vi "CRYCalc Directivity Index.vi"(4 "Weighting curve":string, 6 "Direct_weight":bool caption="Weighting", 7 "Inc(deg.)":i32, 8 "Total Rotation":i32, 9 "Curve Group":string[](array[string]), 10 "Auto Inc":bool caption="Auto Increment", 11 "Curve in":T1={"Name"="", "Curve"=[], "X data"=1, "Y data"=1, "Z data"=1, "X axis"=0, "Y axis"=1, "Z axis"=1, "X unit"="Hz", "Y unit"="", "Z unit"="deg.", "X dB ref"=1.0, "Y dB ref"=1.0, "Z dB ref"=1.0, "single val"=FALSE, "protected"=FALSE, "display X"=TRUE, "display Y"=TRUE, "display Z"=TRUE, "Test Info"="", "Step No."=0, "Plot Settings"={"Color"=0, "Interpolation"=0, "Point Style"=0, "Line Style"=0, "Point Color"=0, "Line Width"=0, "Bar Plot Style"=0, "Fill To"=0}, "AutoProtect"=FALSE} {"Z data" items=["dB", "Lin"]; "X data" items=["dB", "Lin"]; "Y data" items=["dB", "Lin"]; "Z dB ref" format="%.1f"; "Z axis" items=["Log", "Lin"]; "X dB ref" format="%.1f"; "X axis" items=["Log", "Lin"]; "Y axis" items=["Log", "Lin"]; "Y dB ref" format="%.1f"; "Curve"."z" format="%.2f"; "Curve"."y" format="%.2f"; "Curve"."x" format="%.2f"}) -> (3 "Curve out":T1={"Name"="", "Curve"=[], "X data"=1, "Y data"=1, "Z data"=1, "X axis"=0, "Y axis"=1, "Z axis"=1, "X unit"="Hz", "Y unit"="", "Z unit"="deg.", "X dB ref"=1.0, "Y dB ref"=1.0, "Z dB ref"=1.0, "single val"=FALSE, "protected"=FALSE, "display X"=TRUE, "display Y"=TRUE, "display Z"=TRUE, "Test Info"="", "Step No."=0, "Plot Settings"={"Color"=0, "Interpolation"=0, "Point Style"=0, "Line Style"=0, "Point Color"=0, "Line Width"=0, "Bar Plot Style"=0, "Fill To"=0}, "AutoProtect"=FALSE} {"Z data" items=["dB", "Lin"]; "X data" items=["dB", "Lin"]; "Y data" items=["dB", "Lin"]; "Z dB ref" format="%.1f"; "Z axis" items=["Log", "Lin"]; "X dB ref" format="%.1f"; "X axis" items=["Log", "Lin"]; "Y axis" items=["Log", "Lin"]; "Y dB ref" format="%.1f"; "Curve"."z" format="%.2f"; "Curve"."y" format="%.2f"; "Curve"."x" format="%.2f"})   [LabVIEW 2013]
uses:
  Typedef Control/CRYData Cluster.ctl
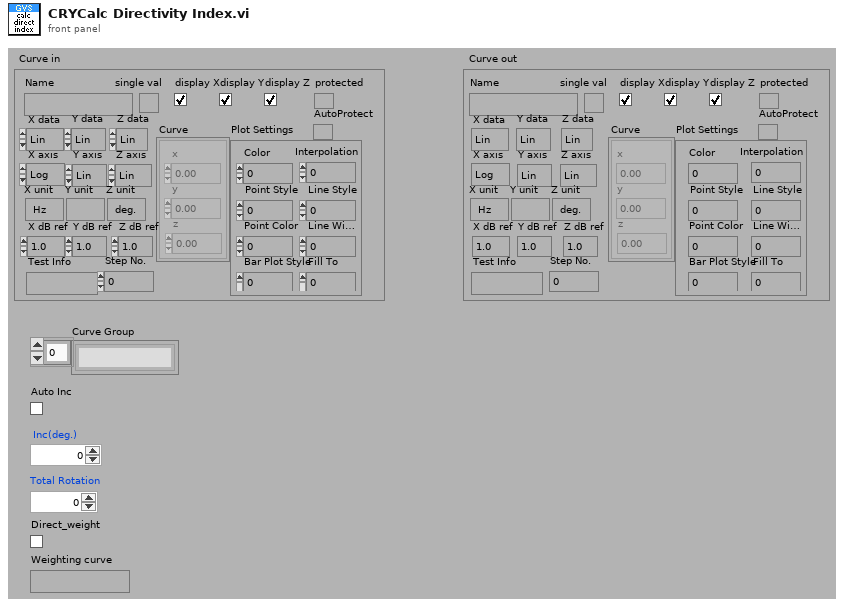
[diagram p1: front panel]
types:
  T1 = typedef "CRYData Cluster.ctl" = cluster{"Name":string, "Curve":cluster{"x":dbl, "y":dbl, "z":dbl}[], "X data":u16, "Y data":u16, "Z data":u16, "X axis":u16, "Y axis":u16, "Z axis":u16, "X unit":string, "Y unit":string, "Z unit":string, "X dB ref":dbl, "Y dB ref":dbl, "Z dB ref":dbl, "single val":bool, "protected":bool, "display X":bool, "display Y":bool, "display Z":bool, "Test Info":string, "Step No.":i32, "Plot Settings":cluster{"Color":u32, "Interpolation":u8, "Point Style":u8, "Line Style":u8, "Point Color":u32, "Line Width":u8, "Bar Plot Style":u8, "Fill To":i16}, "AutoProtect":bool}
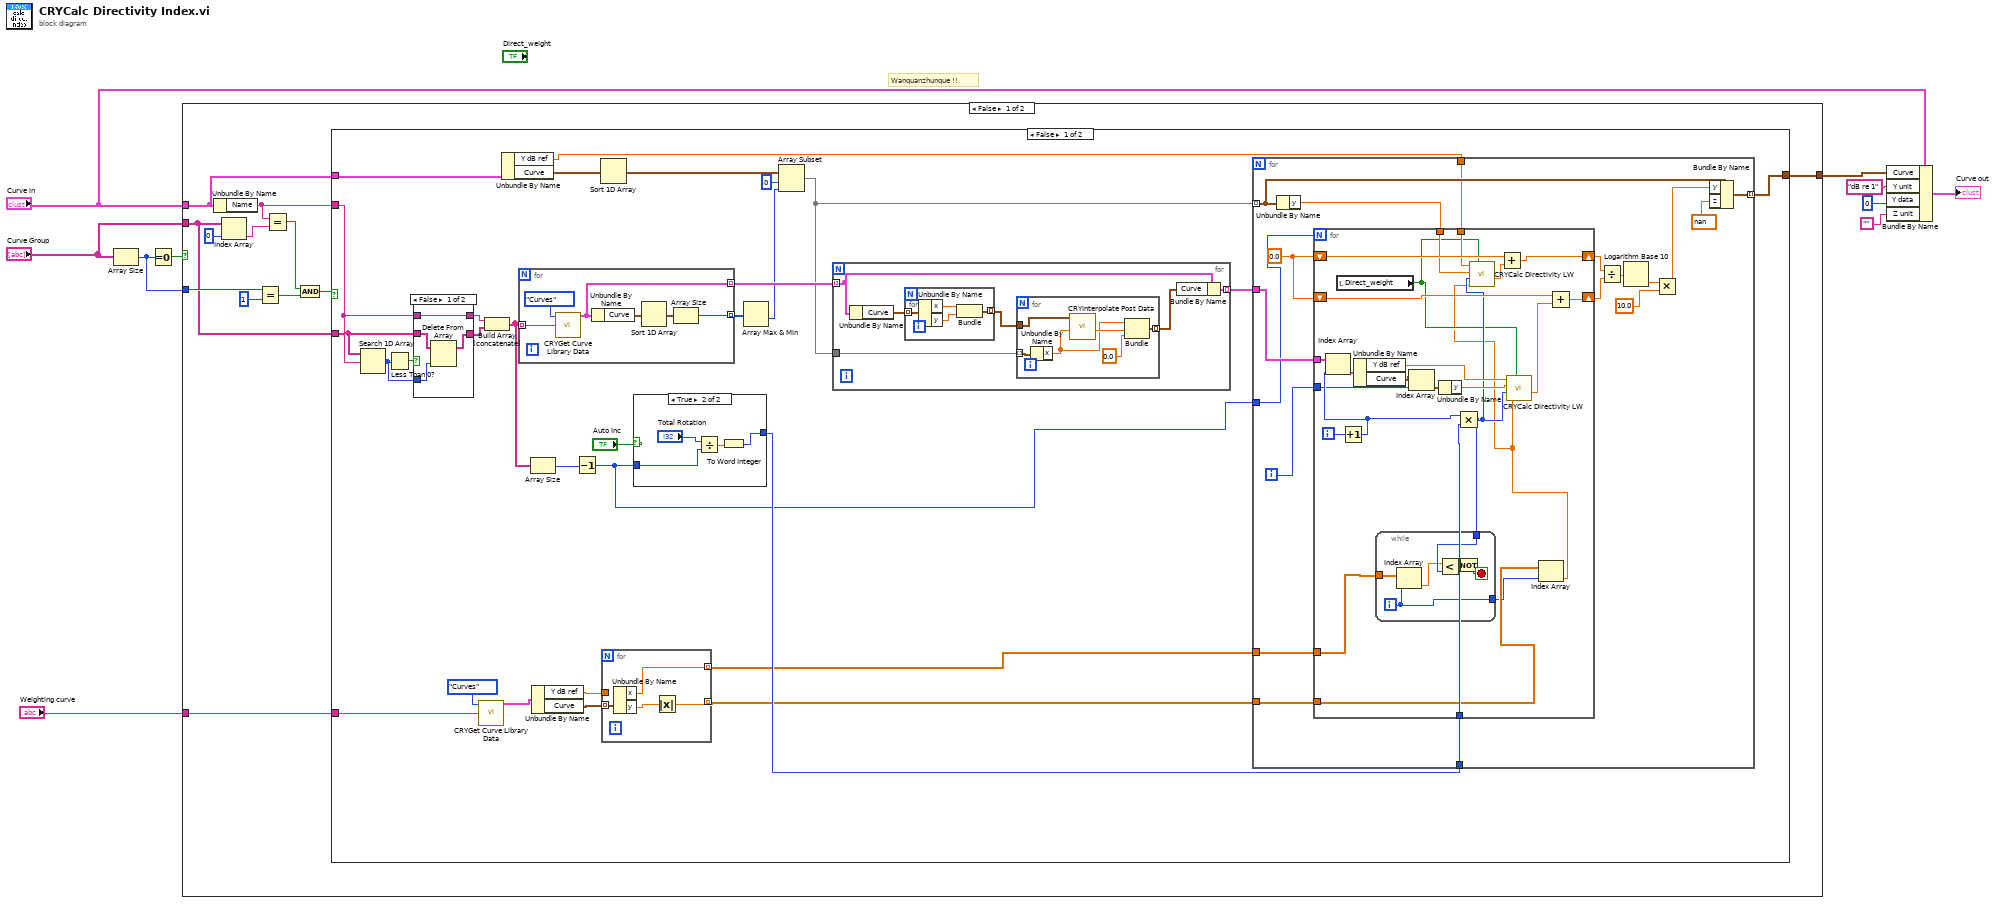
[diagram p0: block diagram]
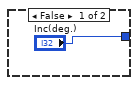
[diagram p2: hidden frame]
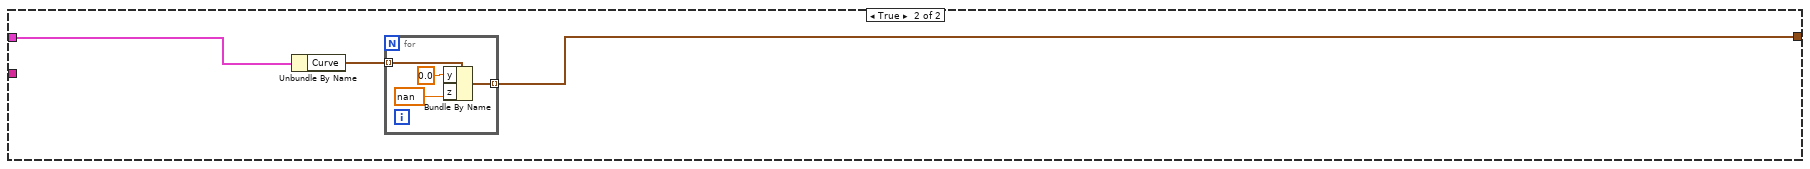
[diagram p4: hidden frame]
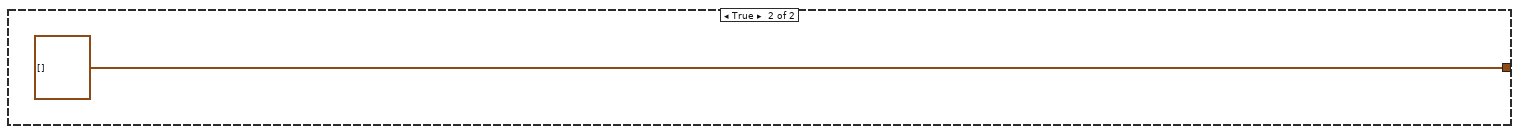
[diagram p5: hidden frame]
diagram:
  # "Wanquanzhunque !!"
  n1 = Array Size(array="Curve Group") -> (size(s)=w5:i32)
  n2 = Equal To 0?(x=w5) -> (x = 0?=w8:bool)
  n3 = case shown="False" w8 {
    tunnel: "Curve in" -> [w17 _]
    tunnel: [w16 cluster{"x":dbl, "y":dbl, "z":dbl}[] [] ("Curve")] -> w6
    tunnel: w5 -> [w22 _]
    tunnel: "Curve Group" -> [w14 _]
    tunnel: "Weighting curve" -> [w11 _]
    frame False {
      n4 = Unbundle By Name(w17) -> ("Name"=w13:string)
      n5 = Index Array(array=w14, index=0) -> (element=w12:string)
      n6 = Equal?(x=w22, y=1) -> (x = y?=w15:bool)
      n7 = Equal?(x=w13, y=w12) -> (x = y?=w19:bool)
      n8 = And(x=w19, y=w15) -> (x .and. y?=w18:bool)
      n9 = case shown="False" w18 {
        tunnel: w17 -> [w51 w139]
        tunnel: [w49 w137] -> w16
        tunnel: w14 -> [w38 _]
        tunnel: w13 -> [w41 _]
        tunnel: w11 -> [w25 _]
        frame False {
          n10 = Search 1D Array(1D array=w38, element=w41) -> (index of element=w37:i32)  [unwired: 1 in]
          n11 = Less Than 0?(x=w37) -> (x < 0?=w42:bool)
          n12 = case shown="False" w42 {
            tunnel: [w64 w66] -> w40
            tunnel: w41 -> [w64 w66]
            tunnel: [w61 w65] -> w39
            tunnel: w38 -> [w63 w65]
            tunnel: w37 -> [w62 _]
            frame False {
              n13 = Delete From Array(array=w63, index=w62) -> (array with subset deleted=w61:string[])  [unwired: 1 in, 1 out]
            }
            frame True {
            }
          }
          n14 = call "CRYGet Curve Library Data.vi"("Type"=enum16{"Curves", "Values", "Results", "WFM"}."Curves", "Data Name"=w25) -> ("Curve"=w27:T1)  [unwired: 4 out]
          n15 = Build Array (concatenate)(w40, w39) -> (w35:string[])
          n16 = Unbundle By Name(w51) -> ("Y dB ref"=w36:dbl, "Curve"=w50:cluster{"x":dbl, "y":dbl, "z":dbl}[])
          n17 = for {
            tunnel: w35 -> [w135] mode=indexing
            tunnel: [w134] -> w45 mode=indexing
            tunnel: [w131] -> w46 mode=indexing
            n18 = call "CRYGet Curve Library Data.vi"("Type"=enum16{"Curves", "Values", "Results", "WFM"}."Curves", "Data Name"=w135) -> ("Curve"=w134:T1)  [unwired: 4 out]
            n19 = Unbundle By Name(w134) -> ("Curve"=w133:cluster{"x":dbl, "y":dbl, "z":dbl}[])
            n20 = Sort 1D Array(array=w133) -> (sorted array=w132:cluster{"x":dbl, "y":dbl, "z":dbl}[])
            n21 = Array Size(array=w132) -> (size(s)=w131:i32)
          }
          n22 = Array Size(array=w35) -> (size(s)=w33:i32)
          n23 = Unbundle By Name(w27) -> ("Y dB ref"=w26:dbl, "Curve"=w28:cluster{"x":dbl, "y":dbl, "z":dbl}[])
          n24 = Decrement(x=w33) -> (x-1=w30:i32)
          n25 = Sort 1D Array(array=w50) -> (sorted array=w48:cluster{"x":dbl, "y":dbl, "z":dbl}[])
          n26 = for {
            tunnel: w28 -> [w55] mode=indexing
            tunnel: w26 -> [_]
            tunnel: [w52] -> w23 mode=indexing
            tunnel: [w54] -> w24 mode=indexing
            n27 = Unbundle By Name(w55) -> ("x"=w54:dbl, "y"=w53:dbl)
            n28 = Absolute Value(x=w53) -> (abs(x)=w52:dbl)
          }
          n29 = case shown="True" "Auto Inc" {
            tunnel: w30 -> [_ w59]
            tunnel: ["Inc(deg.)" w57] -> w31
            frame False {
            }
            frame True {
              n30 = Divide(x="Total Rotation", y=w59) -> (x/y=w58:dbl)
              n31 = To Word Integer(number=w58) -> (16bit integer=w57:i16)
            }
          }
          n32 = Array Max & Min(array=w46) -> (min value=w43:i32)  [unwired: 3 out]
          n33 = Array Subset(array=w48, index=0, length=w43) -> (w44:cluster{"x":dbl, "y":dbl, "z":dbl}[])
          n34 = for {
            tunnel: w45 -> [w70] mode=indexing
            tunnel: [w72] -> w32 mode=indexing
            tunnel: w44 -> [w71]
            n35 = Unbundle By Name(w70) -> ("Curve"=w69:cluster{"x":dbl, "y":dbl, "z":dbl}[])
            n36 = for {
              tunnel: w69 -> [w76] mode=indexing
              tunnel: [w73] -> w68 mode=indexing
              n37 = Unbundle By Name(w76) -> ("x"=w75:dbl, "y"=w74:dbl)
              n38 = Bundle("x"=w75, "y"=w74) -> (w73:cluster{"x":dbl, "y":dbl})  [unwired: 1 in]
            }
            n39 = for {
              tunnel: w71 -> [w82] mode=indexing
              tunnel: w68 -> [w81]
              tunnel: [w77] -> w67 mode=indexing
              n40 = Unbundle By Name(w82) -> ("x"=w79:dbl)
              n41 = call "CRYInterpolate Post Data.vi"("X value"=w79, "Curve in"=w81) -> ("Y value"=w80:dbl)  [unwired: 9 in]
              n42 = Bundle("x"=w79, "Y value"=w80, "x"=0.0) -> (w77:cluster{"x":dbl, "Y value":dbl, "x":dbl})  [unwired: 1 in]
            }
            n43 = Bundle By Name(cluster=w70, "Curve"=w67) -> (w72:T1)
          }
          n44 = for {
            tunnel: w32 -> [w86]
            tunnel: w44 -> [w100] mode=indexing
            tunnel: [w98] -> w49 mode=indexing
            tunnel: w36 -> [w89]
            tunnel: w31 -> [w88]
            tunnel: w30 -> [w85]
            tunnel: w24 -> [w84]
            tunnel: w23 -> [w83]
            i -> [w87]
            w97 = 0.0
            n45 = Unbundle By Name(w100) -> ("y"=w91:dbl)
            n46 = for {
              N: w85 -> [_]
              shift-right: [w124] -> w93
              shift-left: w97 -> [w123]
              shift-right: [w121] -> w92
              shift-left: w97 -> [w120]
              tunnel: w91 -> [w110]
              tunnel: w89 -> [w119]
              tunnel: w88 -> [w118]
              tunnel: w86 -> [w116]
              tunnel: w87 -> [w111]
              tunnel: w84 -> [w106]
              tunnel: w83 -> [w104]
              i -> [w117]
              n47 = local read "Direct_weight"() -> (w103:bool)
              n48 = Increment(x=w117) -> (x+1=w115:i32)
              n49 = Index Array(array=w116, index=w115) -> (element=w114:T1)
              n50 = Unbundle By Name(w114) -> ("Y dB ref"=w107:dbl, "Curve"=w112:cluster{"x":dbl, "y":dbl, "z":dbl}[])
              n51 = Index Array(array=w112, index=w111) -> (element=w113:cluster{"x":dbl, "y":dbl, "z":dbl})
              n52 = Unbundle By Name(w113) -> ("y"=w109:dbl)
              n53 = Multiply(x=w115, y=w118) -> (x*y=w105:i32)
              n54 = while {
                tunnel: w106 -> [w130]
                tunnel: w105 -> [w126]
                tunnel: [w129] -> w101
                i -> [w129]
                stop <- w128 stop-if-true
                n55 = Index Array(array=w130, index=w129) -> (element=w125:dbl)
                n56 = Less?(x=w125, y=w126) -> (x < y?=w127:bool)
                n57 = Not(x=w127) -> (.not. x?=w128:bool)
              }
              n58 = Index Array(array=w104, index=w101) -> (element=w102:dbl)
              n59 = call "CRYCalc Directivity LW.vi"("Direct_weight"=w103, "weight"=w102, "Degree"=w105, "In L(f)"=w110, "Y ref"=w119) -> ("L(f)*W(deg)"=w122:dbl)  [unwired: 6 in]
              n60 = Add(x=w120, y=w122) -> (x+y=w121:dbl)
              n61 = call "CRYCalc Directivity LW.vi"("Direct_weight"=w103, "weight"=w102, "Degree"=w105, "In L(f)"=w109, "Y ref"=w107) -> ("L(f)*W(deg)"=w108:dbl)  [unwired: 6 in]
              n62 = Add(x=w123, y=w108) -> (x+y=w124:dbl)
            }
            n63 = Divide(x=w92, y=w93) -> (x/y=w94:dbl)
            n64 = Logarithm Base 10(1:w94) -> (0:w95:dbl)
            n65 = Multiply(x=w95, y=10.0) -> (x*y=w90:dbl)
            n66 = Bundle By Name(cluster=w100, "y"=w90, "z"=nan) -> (w98:cluster{"x":dbl, "y":dbl, "z":dbl})
          }
        }
        frame True {
          n67 = Unbundle By Name(w139) -> ("Curve"=w138:cluster{"x":dbl, "y":dbl, "z":dbl}[])
          n68 = for {
            tunnel: w138 -> [w143] mode=indexing
            tunnel: [w140] -> w137 mode=indexing
            n69 = Bundle By Name(cluster=w143, "y"=0.0, "z"=nan) -> (w140:cluster{"x":dbl, "y":dbl, "z":dbl})
          }
        }
      }
    }
    frame True {
    }
  }
  n70 = Bundle By Name(cluster="Curve in", "Curve"=w6, "Y unit"="dB re 1", "Y data"=u16 0, "Z unit"="") -> (→"Curve out":T1)
